vi "Get Error Codes.vi"(8 "error in (no error)":errorcluster, 11 "UDP in":refnum<class "UDP.lvclass">) -> (0 "error out":errorcluster, 2 "Error Codes":cluster{"Code":i32, "String":string}[](array[cluster]), 3 "UDP out":refnum<class "UDP.lvclass">)   [LabVIEW 2019, in "Protocols.lvlib" / "UDP.lvclass"]
uses:
  UDP.lvclass
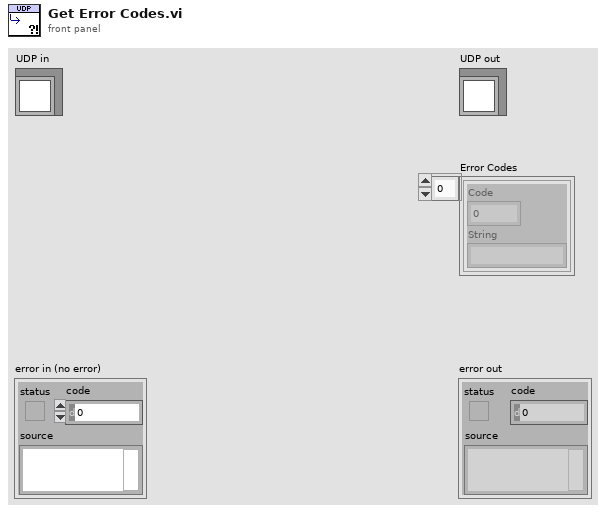
[diagram p1: front panel]
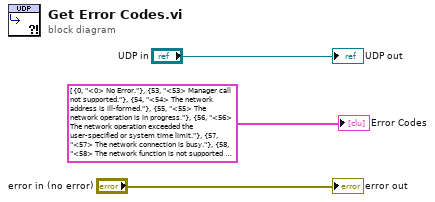
[diagram p0: block diagram]
diagram:
  "error out" <- "error in (no error)"
  "UDP out" <- "UDP in"
  "Error Codes" <- cluster{"Code":i32, "String":string}[] [{"Code"=0, "String"="<0> No Error."}, {"Code"=53, "String"="<53> Manager call not supported."}, {"Code"=54, "String"="<54> The network address is ill-formed."}, {"Code"=55, "String"="<55> The network operation is in progress."}, {"Code"=56, "String"="<56> The network operation exceeded the user-specified or system time limit."}, {"Code"=57, "String"="<57> The network connection is busy."}, {"Code"=58, "String"="<58> The network function is not supported by the system."}, {"Code"=59, "String"="<59> The network is down, unreachable, or has been reset."}, {"Code"=60, "String"="<60> The specified port or network address is currently in use."}, {"Code"=61, "String"="<61> The system could not allocate the necessary memory."}, {"Code"=62, "String"="<62> The system caused the network connection to be aborted."}, {"Code"=63, "String"="<63> The network connection was refused by the server."}, {"Code"=64, "String"="<64> The network connection is not yet established."}, {"Code"=65, "String"="<65> The network connection is already established."}, {"Code"=66, "String"="<66> The network connection was closed by the peer."}, {"Code"=108, "String"="<108> Singlecast connections cannot send to multicast addresses."}, {"Code"=109, "String"="<109> Multicast connections cannot send to singlecast addresses."}, {"Code"=110, "String"="<110> Specified IP address is not in multicast address range."}, {"Code"=111, "String"="<111> Cannot write to read-only multicast connection."}, {"Code"=112, "String"="<112> Cannot read from write-only multicast connection."}, {"Code"=113, "String"="<113> A message sent on a datagram socket was larger than the message buffer, network limit, or the receive buffer was to small."}, {"Code"=127, "String"="<127> The specified socket is not an IPv4 socket."}] ("appended array")
